vi "compare.vi"(5 "control references":T1, 6 "internet error?":bool, 7 "internet version in":string, 8 "error in (no error)":errorcluster, 9 "local error?":bool, 10 "local version in":string, 11 "HelioUpdateMH100803 in":refnum<class "HelioUpdateMH100803.lvclass">) -> (0 "error out":errorcluster, 3 "HelioUpdateMH100803 out":refnum<class "HelioUpdateMH100803.lvclass">, 4 "update out":T2)   [LabVIEW 2010, in "HelioUpdateMH100803.lvclass"]
uses:
  HelioUpdateMH100803.lvclass
  main/labview_source/controls/update_picture.ctl
  main/labview_source/type_definitions/clusters/controls_refs.ctl
  <vilib>/Utility/miscctls.llb/LVPositionTypeDef.ctl
  <vilib>/Utility/miscctls.llb/LVBoundsTypeDef.ctl
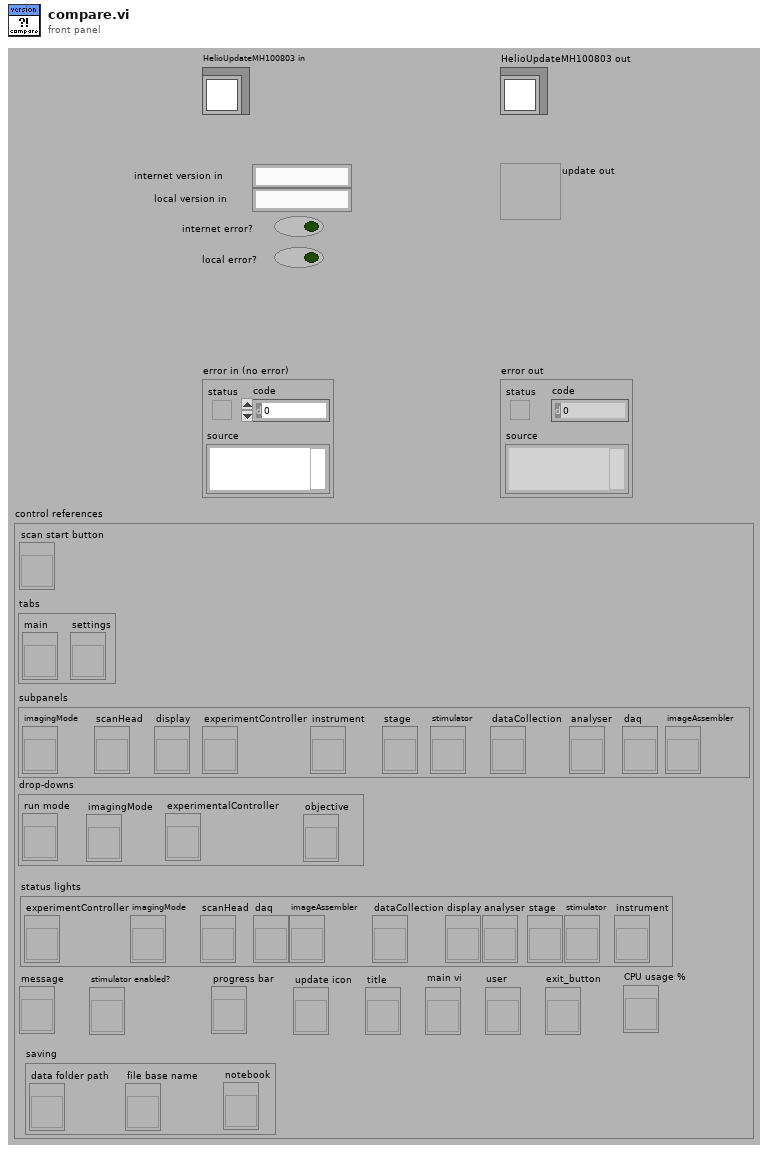
[diagram p1: front panel]
types:
  T1 = typedef "controls_refs.ctl" = cluster{"scan start button":refnum<vi>, "tabs":cluster{"main":refnum<vi>, "settings":refnum<vi>}, "subpanels":cluster{"imagingMode":refnum<vi>, "scanHead":refnum<vi>, "display":refnum<vi>, "experimentController":refnum<vi>, "instrument":refnum<vi>, "stage":refnum<vi>, "stimulator":refnum<vi>, "dataCollection":refnum<vi>, "analyser":refnum<vi>, "daq":refnum<vi>, "imageAssembler":refnum<vi>}, "drop-downs":cluster{"run mode":refnum<vi>, "imagingMode":refnum<vi>, "experimentalController":refnum<vi>, "objective":refnum<vi>}, "status lights":cluster{"experimentController":refnum<vi>, "imagingMode":refnum<vi>, "scanHead":refnum<vi>, "daq":refnum<vi>, "imageAssembler":refnum<vi>, "dataCollection":refnum<vi>, "display":refnum<vi>, "analyser":refnum<vi>, "stage":refnum<vi>, "stimulator":refnum<vi>, "instrument":refnum<vi>}, "message":refnum<vi>, "stimulator enabled?":refnum<vi>, "saving":cluster{"data folder path":refnum<vi>, "file base name":refnum<vi>, "notebook":refnum<vi>}, "progress bar":refnum<vi>, "update icon":refnum<vi>, "title":refnum<vi>, "main vi":refnum<vi>, "user":refnum<vi>, "exit_button":refnum<vi>, "CPU usage %":refnum<vi>}
  T2 = typedef "HelioUpdateMH100803.lvclass/update_picture.ctl" = u16
  T3 = typedef "LVPositionTypeDef.ctl" = cluster{"Left":i32, "Top":i32}
  T4 = typedef "LVBoundsTypeDef.ctl" = cluster{"Width":u32, "Height":u32}
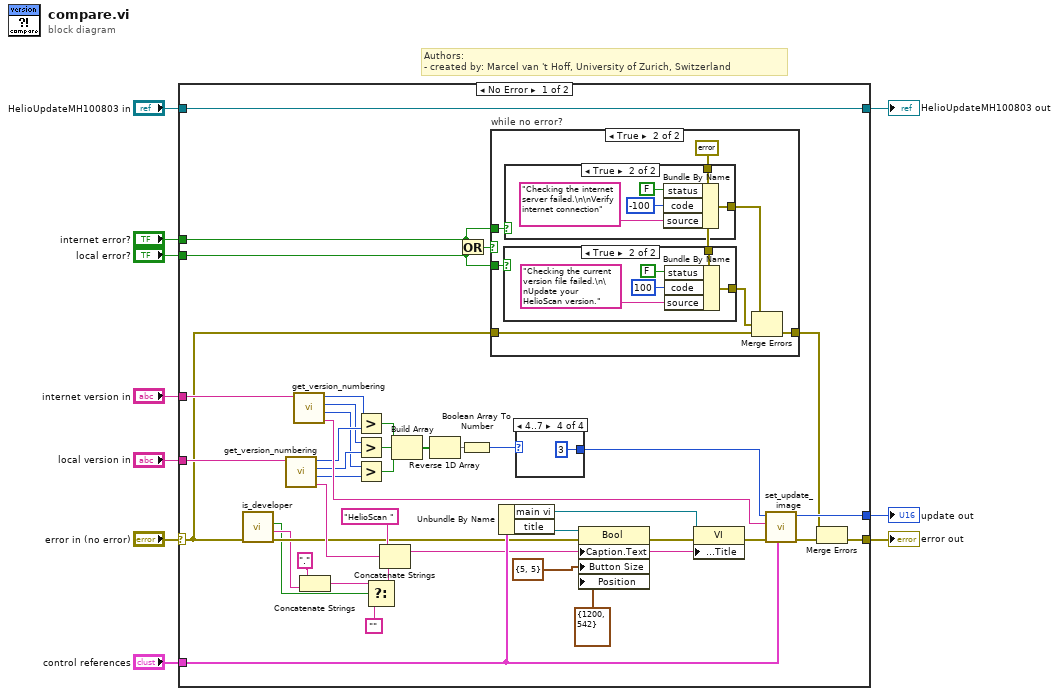
[diagram p0: block diagram]
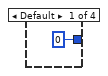
[diagram p2: hidden frame]
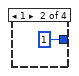
[diagram p3: hidden frame]
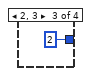
[diagram p4: hidden frame]
diagram:
  # "Authors: \n- created by: Marcel van 't Hoff, University of Zurich, Switzerland"
  n1 = case shown="No Error" "error in (no error)" {
    selector: "error in (no error)" -> [w19 w76]
    tunnel: [w22 w76] -> w9
    tunnel: [w52 w75] -> w7
    tunnel: "HelioUpdateMH100803 in" -> [w52 w75]
    tunnel: "local version in" -> [w41 _]
    tunnel: "internet version in" -> [w40 _]
    tunnel: "internet error?" -> [w50 _]
    tunnel: "local error?" -> [w49 _]
    tunnel: [w48 _] -> w2
    tunnel: "control references" -> [w46 _]
    frame No Error {
      n2 = call "is_developer.vi"("error in (no error)"=w19) -> ("error out"=w18:errorcluster, "svn version number"=w13:string, "is developer?"=w11:bool)  [unwired: 8 in]
      n3 = call "get_version_numbering.vi"("local version in"=w41) -> ("resulting string"=w39:string, "revision out"=w32:i32, "minor out"=w34:i32, "mayor out"=w36:i32)  [unwired: 7 in]
      n4 = call "get_version_numbering.vi"("local version in"=w40) -> ("resulting string"=w38:string, "revision out"=w33:i32, "minor out"=w35:i32, "mayor out"=w37:i32)  [unwired: 7 in]
      n5 = Concatenate Strings("." ("string"), w13) -> (w12:string)
      n6 = Greater?(x=w37, y=w36) -> (0:w29:bool)
      n7 = Greater?(x=w35, y=w34) -> (0:w30:bool)
      n8 = Greater?(x=w33, y=w32) -> (0:w31:bool)
      n9 = Select(t=w12, s=w11, f="") -> (s? t:f=w15:string)
      n10 = Concatenate Strings("HelioScan ", w39, w15) -> (w17:string)
      n11 = Build Array(w29, w30, w31) -> (w28:bool[])
      n12 = Reverse 1D Array(array=w28) -> (reversed array=w26:bool[])
      n13 = Or(x=w50, y=w49) -> (x .or. y?=w51:bool)
      n14 = Boolean Array To Number(Boolean array=w26) -> (number=w27:u32)
      n15 = case "while no error?" shown="True" w51 {
        tunnel: w50 -> [_ w64]
        tunnel: w49 -> [_ w63]
        tunnel: [w57 w60] -> w24
        tunnel: w19 -> [w57 w59]
        frame False {
        }
        frame True {
          w58 = errorcluster {"status"=FALSE, "code"=0, "source"=""} ("error in (no error)")
          n16 = case shown="True" w63 {
            tunnel: w58 -> [_ w69]
            tunnel: [_ w65] -> w61
            frame False {
            }
            frame True {
              n17 = Bundle By Name(cluster=w69, "status"=FALSE, "code"=100, "source"="Checking the current version file failed.\n\nUpdate your HelioScan version." ("message")) -> (w65:errorcluster)
            }
          }
          n18 = case shown="True" w64 {
            tunnel: w58 -> [_ w74]
            tunnel: [_ w70] -> w62
            frame False {
            }
            frame True {
              n19 = Bundle By Name(cluster=w74, "status"=FALSE, "code"=-100, "source"="Checking the internet server failed.\n\nVerify internet connection" ("message")) -> (w70:errorcluster)
            }
          }
          n20 = Merge Errors(w62, w61, w59) -> (w60:errorcluster)
        }
      }
      n21 = Unbundle By Name(w46) -> ("main vi"=w42:refnum<vi>, "title"=w45:refnum<vi>)
      n22 = case shown="4..7" w27 {
        tunnel: [T2 0 ("update in") T2 1 ("update in") T2 2 ("update in") T2 3 ("update in")] -> w21
        frame Default {
        }
        frame 1 {
        }
        frame 2, 3 {
        }
        frame 4..7 {
        }
      }
      n23 = property class="Bool"(reference=w45, error in=w18, "Caption.Text"=w17, "Button Size"=T4 {"Width"=5, "Height"=5}, "Position"=T3 {"Left"=1200, "Top"=542}) -> (error out=w43:errorcluster)  [unwired: 1 out]
      n24 = property class="VI"(reference=w42, error in=w43, "Front Panel.Title"=w17) -> (error out=w25:errorcluster)  [unwired: 1 out]
      n25 = call "set_update_image.vi"("control references"=w46, "error in (no error)"=w25, "internet version in"=w38, "update in"=w21) -> ("error out"=w23:errorcluster, "update out"=w48:T2)  [unwired: 6 in]
      n26 = Merge Errors(w24, w23) -> (w22:errorcluster)
    }
    frame Error {
    }
  }
  "error out" <- w9
  "HelioUpdateMH100803 out" <- w7
  "update out" <- w2
